vi "Get Next Log Engine State.vi"(10 "Log State":T1, 11 "Bus State":T2) -> (3 "Log State":T1)   [LabVIEW 2019, in "CAN Stream Support Workspace Shared.lvlib"]
uses:
  CAN Stream Support Workspace Shared.lvlib
  Types/Host Stream Engine State.ctl
  Types/Host Stream Engine Logging State.ctl
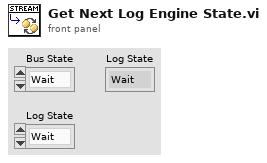
[diagram p1: front panel]
types:
  T1 = typedef "CAN Stream Support Workspace Shared.lvlib/Host Stream Engine Logging State.ctl" = enum8{"Wait", "Logging", "Cleanup", "Exit"}
  T2 = typedef "CAN Stream Support Workspace Shared.lvlib/Host Stream Engine State.ctl" = enum8{"Wait", "Start Stream", "Read Stream", "Stop Stream", "Exit"}
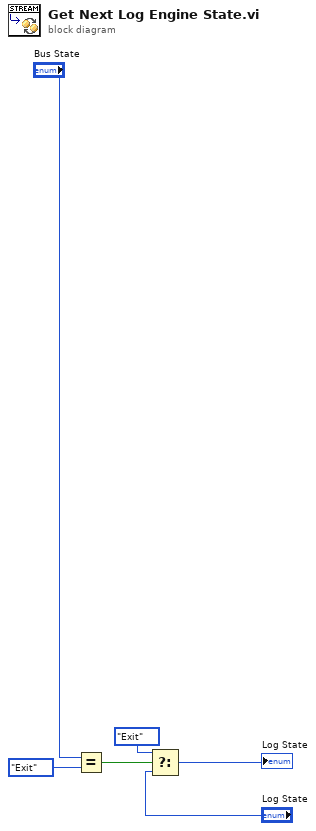
[diagram p0: block diagram]
diagram:
  n1 = Equal?(x="Bus State", y=Host_Stream_Engine_State."Exit") -> (x = y?=w4:bool)
  n2 = Select(t=Host_Stream_Engine_Logging_State."Exit", s=w4, f="Log State") -> (s? t:f=→"Log State":T1)
